vi "Write Generation Status.vi"(0 "generating":bool, 2 "shared":refnum<class "niUSRP Rx Core v1 FPGA.lvclass">=refnum, 5 "waiting for trigger":bool) -> ()   [LabVIEW 2023, in "niUSRP Rx Core v1 FPGA.lvclass"]
doc: "this VI is used to transfer generation statuses across clock domains; from the Generation Loop to the ActiveLED configuration."
uses:
  <instrlib>/niUSRP/Reference FPGA/Rx Core/niUSRP Rx Core v1 FPGA.lvclass
  <vilib>/rvi/DataTransferAndStorage/Container/XNode/niFpgaContainer.xnode
  <vilib>/rvi/DataTransferAndStorage/Register/Emulation/niFpgaRegisterEmulationRefIn.vi
  <instrlib>/niVST/Reference FPGA/FPGA/niUSRP Rx Core v1 FPGA/niUSRP Rx Core v1 FPGA.lvclass
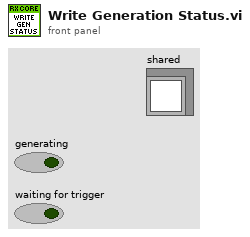
[diagram p1: front panel]
types:
  T1 = typedef "niVST Shared Registers v1 FPGA.lvclass/Shared Registers.ctl" = cluster{"wrapback data":refnum<k21>, "status.gen.generating":refnum<k21>, "status.gen.waiting for trigger":refnum<k21>, "status.acq.in progress":refnum<k21>, "status.acq.waiting for trigger":refnum<k21>}
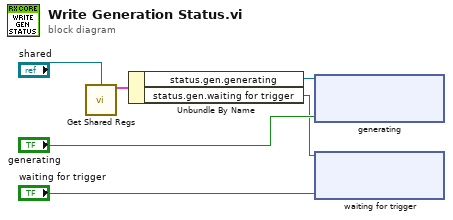
[diagram p0: block diagram]
diagram:
  n1 = call-dynamic "Get Shared Regs.vi"("shared"="shared") -> ("shared regs"=w2:T1)  [unwired: 14 in]
  n2 = Unbundle By Name(w2) -> ("status.gen.generating"=w6:refnum<k21>, "status.gen.waiting for trigger"=w4:refnum<k21>)
  n3 = xnode "generating"("Data"="generating", "Register In"=w6) -> ()  [unwired: 1 out]
  n4 = xnode "waiting for trigger"("Data"="waiting for trigger", "Register In"=w4) -> ()  [unwired: 1 out]
